vi "Read Ref Value.vi"(8 "error in (no error)":errorcluster, 11 "BetterMultiListboxHandle in":refnum<class "BetterMultiListboxHandle.lvclass">) -> (0 "error out":errorcluster, 2 "Value":i32[](array[numeric]), 3 "BetterMultiListboxHandle out":refnum<class "BetterMultiListboxHandle.lvclass">)   [LabVIEW 2020, in "BetterDragAndDrop.lvlib" / "BetterMultiListboxHandle.lvclass"]
uses:
  BetterMultiListboxHandle.lvclass
  BetterMultiListboxHandle.lvclass/BetterMultiListboxHandle.ctl
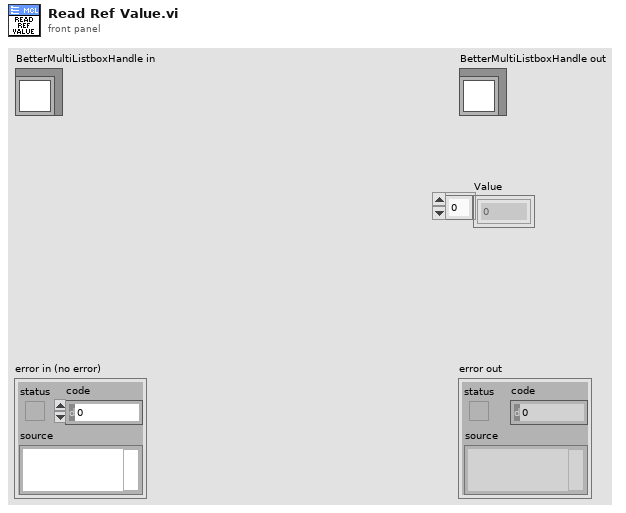
[diagram p1: front panel]
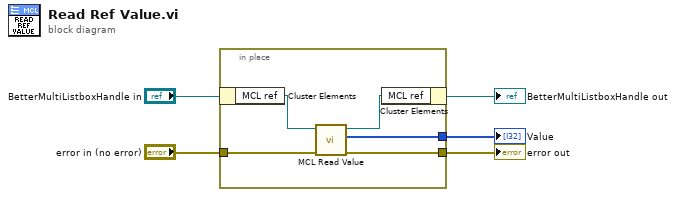
[diagram p0: block diagram]
diagram:
  n1 = in-place {
    in-place-border: "error in (no error)" -> [w6]
    in-place-border: [w7] -> w3
    in-place-border: [w8] -> w1
    n2 = in-place-cluster #1("BetterMultiListboxHandle in") -> ("MCL ref"=w10:refnum<vi>)
    n3 = call "MCL Read Value.vi"("error in (no error)"=w6, "MCL Ref (generic)"=w10) -> ("error out"=w7:errorcluster, "Value"=w8:i32[], "MCL Ref (generic)"=w9:refnum<vi>)  [unwired: 7 in]
    n4 = in-place-cluster #1("MCL ref"=w9) -> (→"BetterMultiListboxHandle out":refnum<class "BetterMultiListboxHandle.lvclass">)
  }
  "error out" <- w3
  "Value" <- w1
